vi "Config Voltage Scan.vi"(5 "Method (Discrete)":i32(ring) items=["Discrete", "Log10", "Log2", "Linear"], 6 "Delta (1)":dbl=1.0 min=-230.0 max=230.0 format="%#_6f", 7 "Coupling (0)":i32 min=0 max=3, 8 "error in":errorcluster, 9 "Ceiling (15)":dbl=15.0 min=0.0003 max=15.0, 10 "Floor (0.03)":dbl=0.03 min=0.0003 max=15.0, 11 "VISA resource name":refnum<visa-resource-name>) -> (0 "error out":errorcluster, 3 "VISA resource name out":refnum<visa-resource-name>)   [LabVIEW 2017, in "Andeen-Hagerling 2700.lvlib"]
doc: "Establishes the position of highest voltage scan within the multidimensional parameter scan system. Also sets the range of highest voltage parameter, Voltage, used during the scan as well as the direction in which the Voltage is changed each time a scan measurement is to be taken."
uses:
  Andeen-Hagerling 2700.lvlib
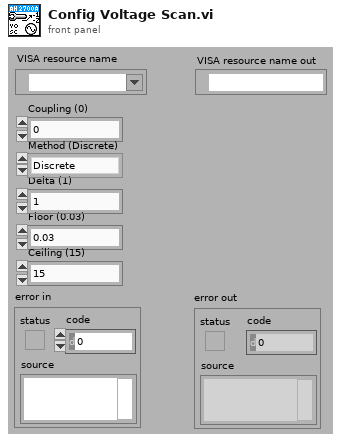
[diagram p1: front panel]
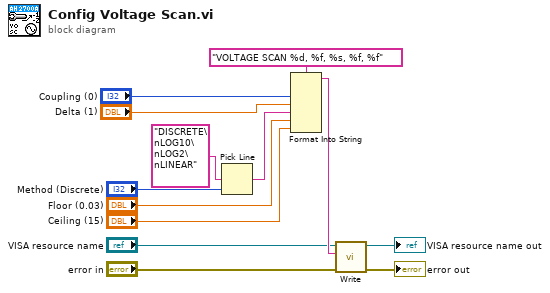
[diagram p0: block diagram]
diagram:
  n1 = Pick Line(multi-line string="DISCRETE\nLOG10\nLOG2\nLINEAR", line index="Method (Discrete)") -> (output string=w3:string)  [unwired: 1 in]
  n2 = Format Into String(format string="VOLTAGE SCAN %d, %f, %s, %f, %f", "Coupling (0)", "Delta (1)", w3, "Floor (0.03)", "Ceiling (15)") -> (resulting string=w11:string)  [unwired: 2 in, 1 out]
  n3 = call "Write.vi"("error in"="error in", "command"=w11, "VISA resource name"="VISA resource name") -> ("error out"=→"error out":errorcluster, "VISA resource name out"=→"VISA resource name out":refnum<visa-resource-name>)  [unwired: 7 in]
